vi "FakeBaseStation (standalone).vi"(0 "Simulated Satellite Data":T1={"Position Array"=[[10, 100], [500, 1000], [90, 270]], "Target Names"=["R", "G", "B", "Q", "R", "S", "T"]}, 1 "STOP":bool) -> (2 "Running?":bool, 3 "Data sent":string, 4 "error out":errorcluster)   [LabVIEW 2012]
panel:
  out "Example Data Sent (data rec'd)":string="$,G,274,67,B,245,67,R,255,42,N,282,44,S,14,5,395\r"
  # "SIMULATED BASE STATION"
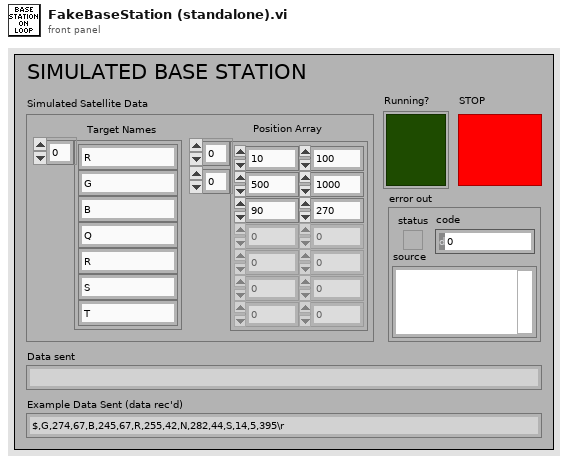
[diagram p1: front panel]
types:
  T1 = cluster{"Position Array":i32[][], "Target Names":string[]}
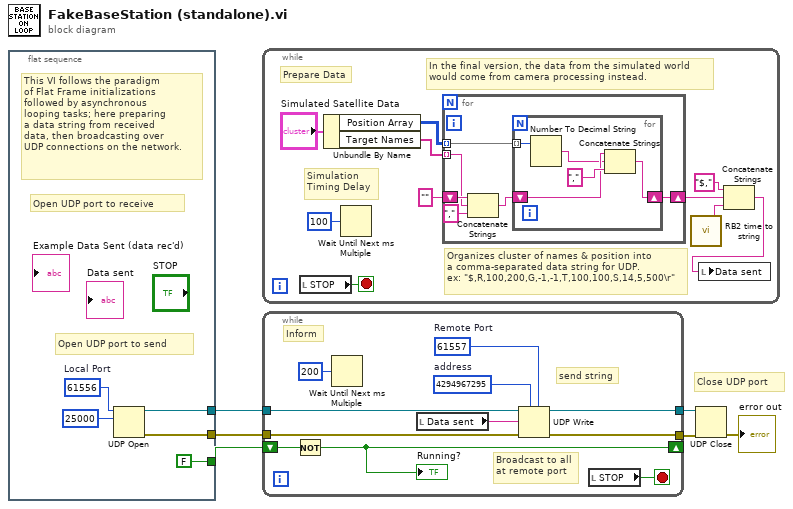
[diagram p0: block diagram]
diagram:
  # "Close UDP port"
  n1 = flat-sequence {
    tunnel: [w9] -> w4
    tunnel: [w8] -> w3
    tunnel: [FALSE] -> w1
    frame #0 {
      w11 = u16 61556  # Local Port
      # "This VI follows the paradigm\nof Flat Frame initializations\nfollowed by asynchronous\nlooping tasks; here preparing\na data string from received\ndata, then broadcasting over\nUDP connections on the network."
      # "Open UDP port to send"
      # "Open UDP port to receive"
      n2 = UDP Open(9:25000 ("timeout ms (25000)"), 11:w11) -> (port=w9:refnum<k16>, 0:w8:errorcluster)  [unwired: 1 in, 3 out]
    }
  }
  n3 = while {
    stop <- w21 stop-if-true
    # "Organizes cluster of names & position into\na comma-separated data string for UDP.\nex: \"$,R,100,200,G,-1,-1,T,100,100,S,14,5,500\\r\""
    # "In the final version, the data from the simulated world\nwould come from camera processing instead."
    # "Simulation\nTiming Delay"
    # "Prepare Data"
    n4 = local read "STOP"() -> (w21:bool)
    n5 = Unbundle By Name("Simulated Satellite Data") -> ("Position Array"=w17:i32[][], "Target Names"=w16:string[])
    n6 = Wait Until Next ms Multiple(millisecond multiple=u32 100) -> ()  [unwired: 1 out]
    n7 = for {
      shift-right: [w26] -> w14
      shift-left: "" -> [w24]
      tunnel: w17 -> [w27] mode=indexing
      tunnel: w16 -> [w23] mode=indexing
      n8 = Concatenate Strings(w24, w23, "," ("string")) -> (w22:string)
      n9 = for {
        shift-right: [w30] -> w26
        shift-left: w22 -> [w31]
        tunnel: w27 -> [w29] mode=indexing
        n10 = Number To Decimal String(number=w29) -> (decimal integer string=w28:string)  [unwired: 1 in]
        n11 = Concatenate Strings(w31, w28, "," ("string")) -> (w30:string)
      }
    }
    n12 = call "RB2 time to string.vi"() -> ("time string"=w12:string)  [unwired: 1 in]
    n13 = Concatenate Strings("$," ("string"), w14, w12) -> (w15:string)
    n14 = local write "Data sent"(w15) -> ()
  }
  n15 = while {
    tunnel: w4 -> [w43]
    tunnel: w3 -> [w42]
    tunnel: [w41] -> w6
    tunnel: [w40] -> w5
    shift-right: [w33] -> _
    shift-left: w1 -> [w34]
    stop <- w36 stop-if-true
    w39 = u16 61557  # Remote Port
    w38 = u32 4294967295  # address
    # "Inform"
    # "send string"
    # "Broadcast to all\nat remote port"
    n16 = Not(x=w34) -> (.not. x?=w33:bool)
    "Running?" <- w33
    n17 = Wait Until Next ms Multiple(millisecond multiple=u32 200) -> ()  [unwired: 1 out]
    n18 = local read "Data sent"() -> (w37:string)
    n19 = UDP Write(address=w38, port or service name=w39, connection ID=w43, data in=w37, 8:w42) -> (error out=w41:errorcluster, 3:w40:refnum<k16>)  [unwired: 1 out]
    n20 = local read "STOP"() -> (w36:bool)
  }
  n21 = UDP Close(connection ID=w5, 8:w6) -> (error out=→"error out":errorcluster)  [unwired: 1 out]
